vi "verify parameters.vi"(8 "error in (no error)":errorcluster, 11 "Channel in":refnum<class "Channel.lvclass">) -> (0 "error out":errorcluster, 3 "Channel out":refnum<class "Channel.lvclass">)   [LabVIEW 2018, in "Channel.lvclass"]
uses:
  Channel.lvclass
  Channel.lvclass/Channel.ctl
  Simulated_CCD_Camera/Simulated_CCD_Camera.lvclass/Simulated_CCD_Camera.ctl
  Simulated_CCD_Camera/Simulated_CCD_Camera.lvclass
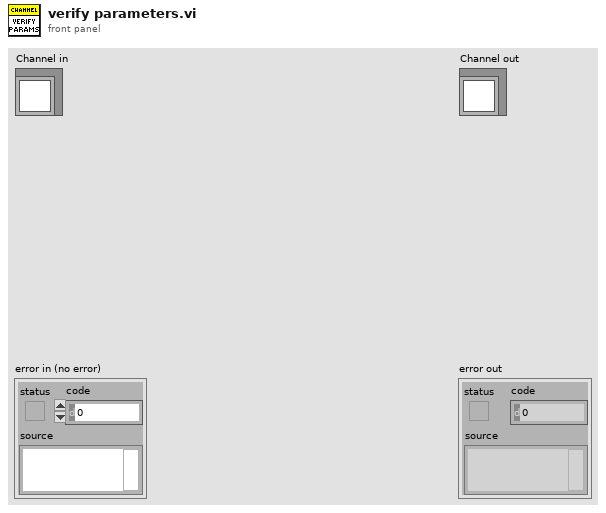
[diagram p1: front panel]
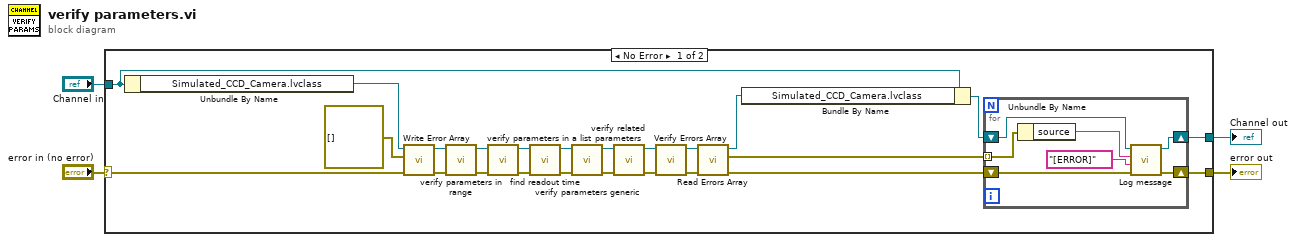
[diagram p0: block diagram]
diagram:
  n1 = case shown="No Error" "error in (no error)" {
    selector: "error in (no error)" -> [w21 w37]
    tunnel: [w15 w37] -> w3
    tunnel: [w16 w36] -> w1
    tunnel: "Channel in" -> [w19 w36]
    frame No Error {
      n2 = Unbundle By Name(w19) -> ("Simulated_CCD_Camera.lvclass"=w20:refnum<class "Simulated_CCD_Camera.lvclass">)
      n3 = call "Write Error Array.vi"("error in (no error)"=w21, "Errors array"=errorcluster[] [], "Simulated_CCD_Camera in"=w20) -> ("error out"=w27:errorcluster, "Simulated_CCD_Camera out"=w28:refnum<class "Simulated_CCD_Camera.lvclass">)  [unwired: 7 in]
      n4 = call "verify parameters in range.vi"("error in (no error)"=w27, "Simulated_CCD_Camera in"=w28) -> ("error out"=w10:errorcluster, "Simulated_CCD_Camera out"=w9:refnum<class "Simulated_CCD_Camera.lvclass">)  [unwired: 8 in]
      n5 = call "verify parameters in a list.vi"("error in (no error)"=w10, "Simulated_CCD_Camera in"=w9) -> ("error out"=w8:errorcluster, "Simulated_CCD_Camera out"=w5:refnum<class "Simulated_CCD_Camera.lvclass">)  [unwired: 8 in]
      n6 = call "find readout time.vi"("error in (no error)"=w8, "Simulated_CCD_Camera in"=w5) -> ("error out"=w7:errorcluster, "Simulated_CCD_Camera out"=w6:refnum<class "Simulated_CCD_Camera.lvclass">)  [unwired: 8 in]
      n7 = call "verify parameters generic.vi"("error in (no error)"=w7, "Simulated_CCD_Camera in"=w6) -> ("error out"=w12:errorcluster, "Simulated_CCD_Camera out"=w11:refnum<class "Simulated_CCD_Camera.lvclass">)  [unwired: 8 in]
      n8 = call "verify related parameters.vi"("error in (no error)"=w12, "Simulated_CCD_Camera in"=w11) -> ("error out"=w24:errorcluster, "Simulated_CCD_Camera out"=w25:refnum<class "Simulated_CCD_Camera.lvclass">)  [unwired: 8 in]
      n9 = call "Verify Errors Array.vi"("error in (no error)"=w24, "Simulated_CCD_Camera in"=w25) -> ("error out"=w22:errorcluster, "Simulated_CCD_Camera out"=w23:refnum<class "Simulated_CCD_Camera.lvclass">)  [unwired: 7 in, 1 out]
      n10 = call "Read Errors Array.vi"("error in (no error)"=w22, "Simulated_CCD_Camera in"=w23) -> ("error out"=w14:errorcluster, "Errors array"=w13:errorcluster[], "Simulated_CCD_Camera out"=w18:refnum<class "Simulated_CCD_Camera.lvclass">)  [unwired: 7 in]
      n11 = Bundle By Name(cluster=w19, "Simulated_CCD_Camera.lvclass"=w18) -> (w17:refnum<class "Channel.lvclass">)
      n12 = for {
        shift-right: [w34] -> w16
        shift-left: w17 -> [w35]
        shift-right: [w33] -> w15
        shift-left: w14 -> [w32]
        tunnel: w13 -> [w31] mode=indexing
        n13 = Unbundle By Name(w31) -> ("source"=w30:string)
        n14 = call "Log message.vi"("error in (no error)"=w32, "message type"="[ERROR]", "String"=w30, "Channel in"=w35) -> ("error out"=w33:errorcluster, "Channel out"=w34:refnum<class "Channel.lvclass">)  [unwired: 6 in]
      }
    }
    frame Error {
    }
  }
  "error out" <- w3
  "Channel out" <- w1
